vi "ADCS.UnlockECUSecurity.vi"(6 "Diagnostic Protocol":T3, 7 "Addon Name":string, 8 "error in (no error)":errorcluster, 9 "MasterKey":string, 10 "Security":T1={"Type"=enum."None", "Source DLL Path"=path "", "Target DLL Path"=path "", "Security Level"=1, "Static Master Key"="", "Max Key Length"=1, "Host IP Address"="", "ECU  Variant"=0, "Optional Parameter"=0}, 11 "diag ref in":T4={"Diag CAN Handle"=0, "Transport Protocol"=enum."ISO TP - Normal Mode", "Receive Address Extension"=0, "Transmit Address Extension"=0, "Receive CAN Id"=0, "Transmit CAN Id"=0, "Log Frames ?"=FALSE, "My TP Address"=0, "Other TP Address"=0, "T1"=0, "T2"=0, "T3"=0, "T4"=0, "Tx SN"=0, "Block Size"=0, "Rx SN"=0, "VW TP Initialized?"=FALSE, "Tx block no"=0, "baud rate"=0, "Interface"="", "Channel Diag CAN Handle"=0, "UDP Connection ID"=refnum, "TCP Connection ID"=refnum, "Target IP Addr"=0, "Source Address"=0, "Target Address"=0, "Send Header NACK?"=FALSE, "DLL Handle"=0, "NAD"=0, "Time Stamp read first"=0.0, "Time Stamp read last"=0.0, "Time Stamp write first"=0.0, "Time Stamp write last"=0.0, "Time Stamp write"=0.0, "Time Stamp read"=0.0, " I/O Mode"=0, "FD Baudrate"=0, "TX_DL"=8, "RX_DL"=8, "DoIP Protocol Version"=1, " Selected I/O Mode"=0, "TesterPresent Counter"=0, "TesterPresent Limit"=0, "TesterPresent Tick[ms]"=10, "TesterPresent RequireResponse?"=FALSE, "TesterPresent Stored Ref?"=FALSE, "TesterPresent Message"=[], "TesterPresent Task Handle"=0, "TesterPresent Semaphore"=refnum, "Response Plausibility Check"=1, "Default Version?"=TRUE, "Diagostic Globals"={"Timeout FC (Bs)"=250, "Timeout CF (Cr)"=250, "Timeout Diag Command"=1000, "Receive Block Size (BS)"=0, "Wait Time CF (STmin)"=5, "Max Waits (N_WFTmax)"=10, "Waits to Send (N_WAIT)"=0, "Time between Waits (TW)"=25, "Fill CAN Frames?"=TRUE, "Fill Byte"=255, "Invalid Response as Error?"=FALSE, "Max RspPending Count"=5, "VWTP Command Timeout"=50, "Transport Protocol"=enum."Diagnostics on IP", "Diag CAN Handle"=0, "DLL Handle"=0, "Timeout RspPending"=1000}, "Session-based Properties?"=FALSE} {"Diagostic Globals"."Fill Byte" format="%x"; "TesterPresent Message" format="%.0x"; "Selected I/O Mode" items=["CAN", "CAN FD", "CAN FD+BRS", "ECU Determined"]; "DoIP Protocol Version" items=["2010"=1, "2012"=2]; "RX_DL" items=["8"=8, "12"=12, "16"=16, "20"=20, "24"=24, "32"=32, "48"=48, "64"=64]; "TX_DL" items=["8"=8, "12"=12, "16"=16, "20"=20, "24"=24, "32"=32, "48"=48, "64"=64]; "I/O Mode" items=["CAN", "CAN FD", "CAN FD+BRS", "Not yet determined"]}) -> (0 "error out":errorcluster, 1 "success?":bool, 3 "diag ref out":T4={"Diag CAN Handle"=0, "Transport Protocol"=enum."ISO TP - Normal Mode", "Receive Address Extension"=0, "Transmit Address Extension"=0, "Receive CAN Id"=0, "Transmit CAN Id"=0, "Log Frames ?"=FALSE, "My TP Address"=0, "Other TP Address"=0, "T1"=0, "T2"=0, "T3"=0, "T4"=0, "Tx SN"=0, "Block Size"=0, "Rx SN"=0, "VW TP Initialized?"=FALSE, "Tx block no"=0, "baud rate"=0, "Interface"="", "Channel Diag CAN Handle"=0, "UDP Connection ID"=refnum, "TCP Connection ID"=refnum, "Target IP Addr"=0, "Source Address"=0, "Target Address"=0, "Send Header NACK?"=FALSE, "DLL Handle"=0, "NAD"=0, "Time Stamp read first"=0.0, "Time Stamp read last"=0.0, "Time Stamp write first"=0.0, "Time Stamp write last"=0.0, "Time Stamp write"=0.0, "Time Stamp read"=0.0, " I/O Mode"=0, "FD Baudrate"=0, "TX_DL"=8, "RX_DL"=8, "DoIP Protocol Version"=1, " Selected I/O Mode"=0, "TesterPresent Counter"=0, "TesterPresent Limit"=0, "TesterPresent Tick[ms]"=10, "TesterPresent RequireResponse?"=FALSE, "TesterPresent Stored Ref?"=FALSE, "TesterPresent Message"=[], "TesterPresent Task Handle"=0, "TesterPresent Semaphore"=refnum, "Response Plausibility Check"=1, "Default Version?"=TRUE, "Diagostic Globals"={"Timeout FC (Bs)"=250, "Timeout CF (Cr)"=250, "Timeout Diag Command"=1000, "Receive Block Size (BS)"=0, "Wait Time CF (STmin)"=5, "Max Waits (N_WFTmax)"=10, "Waits to Send (N_WAIT)"=0, "Time between Waits (TW)"=25, "Fill CAN Frames?"=TRUE, "Fill Byte"=255, "Invalid Response as Error?"=FALSE, "Max RspPending Count"=5, "VWTP Command Timeout"=50, "Transport Protocol"=enum."Diagnostics on IP", "Diag CAN Handle"=0, "DLL Handle"=0, "Timeout RspPending"=1000}, "Session-based Properties?"=FALSE} {"Diagostic Globals"."Fill Byte" format="%x"; "TesterPresent Message" format="%.0x"; "Selected I/O Mode" items=["CAN", "CAN FD", "CAN FD+BRS", "ECU Determined"]; "DoIP Protocol Version" items=["2010"=1, "2012"=2]; "RX_DL" items=["8"=8, "12"=12, "16"=16, "20"=20, "24"=24, "32"=32, "48"=48, "64"=64]; "TX_DL" items=["8"=8, "12"=12, "16"=16, "20"=20, "24"=24, "32"=32, "48"=48, "64"=64]; "I/O Mode" items=["CAN", "CAN FD", "CAN FD+BRS", "Not yet determined"]})   [LabVIEW 2019, in "Diagnostics Addon Engine.lvlib"]
uses:
  Diagnostics Addon Engine.lvlib
  <vilib>/Automotive Diagnostic Command Set/Diagnostic Transport.llb/Diag Reference.ctl
  <vilib>/Automotive Diagnostic Command Set/Diagnostic Transport.llb/Transport Protocol Selector.ctl
  <vilib>/Automotive Diagnostic Command Set/Diagnostic Transport.llb/DoIP Protocol Version.ctl
  <vilib>/Automotive Diagnostic Command Set/Diagnostic Transport.llb/Diag Globals.ctl
  Addon Shared/Types/Protocol.ctl
  Addon Shared/Types/Security.ctl
  Addon Shared/Types/Security.Type.ctl
  <vilib>/NI/STM/Write Meta Data.vi
  <vilib>/NI/STM/TCP/Write Meta Data (TCP Ref).vi
  <vilib>/NI/STM/Get Connection Reference.vi
  <vilib>/NI/STM/TCP/Get Connection Reference (TCP).vi
  <vilib>/Automotive Diagnostic Command Set/Diagnostic Transport.llb/Diagnostic Service.vi
  <vilib>/Automotive Diagnostic Command Set/Diagnostic Transport.llb/Apply Success Failure Error.vi
  <vilib>/NI/STM/TCP/Write Meta Data (TCP Clst).vi
  <vilib>/NI/NI VeriStand Addon Network Comm/Shared/Comm Send and Receive.vi
  <vilib>/Utility/error.llb/Error Cluster From Error Code.vi
  <vilib>/Utility/SystemLogging/Write to System Log.vi
  Support Libraries/GMLAN/_SubVIs/SecurityAccess_requestSeed.vi
  Support Libraries/GMLAN/_SubVIs/SecurityAccess_sendKey.vi
  Support Libraries/GMLAN/GMLAN.lvlib
  <vilib>/addons/Automotive Diagnostic Command Set/NI_Automotive Diagnostic Command Set.lvlib
  Addon Shared/Diagnostics Addon Shared.lvlib
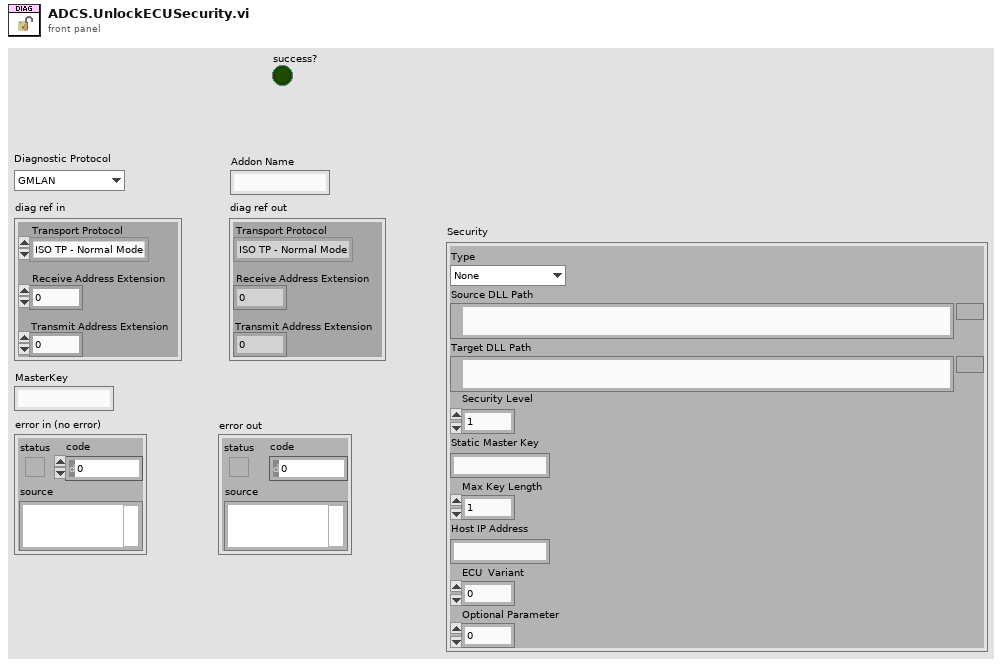
[diagram p1: front panel]
types:
  T1 = typedef "Diagnostics Addon Shared.lvlib/Security.ctl" = cluster{"Type":T2, "Source DLL Path":path, "Target DLL Path":path, "Security Level":u32, "Static Master Key":string, "Max Key Length":u32, "Host IP Address":string, "ECU  Variant":i8, "Optional Parameter":i8}
  T2 = typedef "Diagnostics Addon Shared.lvlib/Security.Type.ctl" = enum16{"None", "SeedKey DLL", "MasterKey (Channel)", "MasterKey (Static)", "SeedKey DLL (Windows)"}
  T3 = typedef "Diagnostics Addon Shared.lvlib/Protocol.ctl" = enum16{"GMLAN", "KWP-2000", "UDS", "User-Defined"}
  T4 = typedef "NI_Automotive Diagnostic Command Set.lvlib/Diag Reference.ctl" = cluster{"Diag CAN Handle":u32, "Transport Protocol":T5, "Receive Address Extension":u8, "Transmit Address Extension":u8, "Receive CAN Id":u32, "Transmit CAN Id":u32, "Log Frames ?":bool, "My TP Address":u8, "Other TP Address":u8, "T1":u16, "T2":u16, "T3":u16, "T4":u16, "Tx SN":u8, "Block Size":u8, "Rx SN":u8, "VW TP Initialized?":bool, "Tx block no":u8, "baud rate":u64, "Interface":string, "Channel Diag CAN Handle":u32, "UDP Connection ID":refnum<k16>, "TCP Connection ID":refnum<k5>, "Target IP Addr":u32, "Source Address":u16, "Target Address":u16, "Send Header NACK?":bool, "DLL Handle":u32, "NAD":u8, "Time Stamp read first":dbl, "Time Stamp read last":dbl, "Time Stamp write first":dbl, "Time Stamp write last":dbl, "Time Stamp write":dbl, "Time Stamp read":dbl, " I/O Mode":u32, "FD Baudrate":u64, "TX_DL":u16, "RX_DL":u16, "DoIP Protocol Version":T6, " Selected I/O Mode":u32, "TesterPresent Counter":u32, "TesterPresent Limit":u32, "TesterPresent Tick[ms]":i32, "TesterPresent RequireResponse?":bool, "TesterPresent Stored Ref?":bool, "TesterPresent Message":u8[], "TesterPresent Task Handle":i32, "TesterPresent Semaphore":T7, "Response Plausibility Check":u32, "Default Version?":bool, "Diagostic Globals":T8, "Session-based Properties?":bool}
  T5 = typedef "NI_Automotive Diagnostic Command Set.lvlib/Transport Protocol Selector.ctl" = enum16{"ISO TP - Normal Mode", "ISO TP - Mixed Mode", "VW TP 2.0", "Diagnostics on IP", "ISO TP LIN"}
  T6 = typedef "NI_Automotive Diagnostic Command Set.lvlib/DoIP Protocol Version.ctl" = u8
  T7 = typedef "Semaphore RefNum" = refnum<k1>
  T8 = typedef "NI_Automotive Diagnostic Command Set.lvlib/Diag Globals.ctl" = cluster{"Timeout FC (Bs)":u32, "Timeout CF (Cr)":u32, "Timeout Diag Command":u32, "Receive Block Size (BS)":u8, "Wait Time CF (STmin)":u8, "Max Waits (N_WFTmax)":u8, "Waits to Send (N_WAIT)":i32, "Time between Waits (TW)":u32, "Fill CAN Frames?":bool, "Fill Byte":u32, "Invalid Response as Error?":bool, "Max RspPending Count":u32, "VWTP Command Timeout":u32, "Transport Protocol":T5, "Diag CAN Handle":u32, "DLL Handle":u32, "Timeout RspPending":u32}
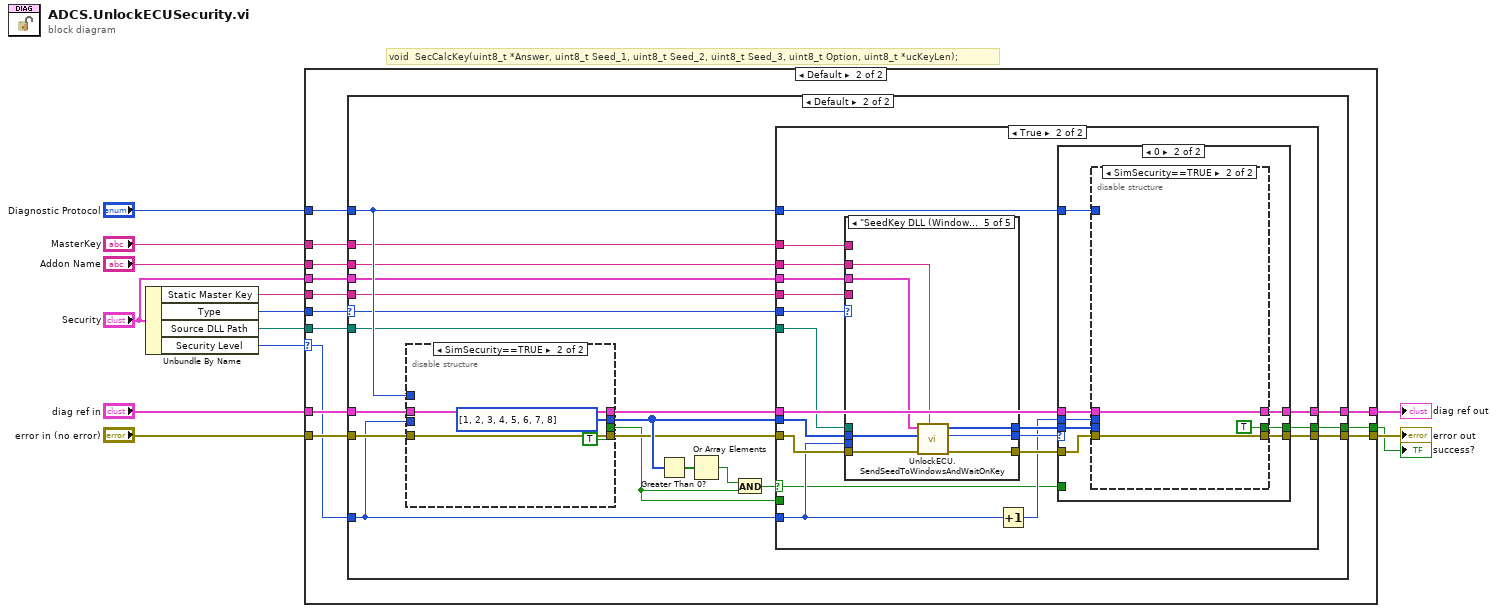
[diagram p0: block diagram]
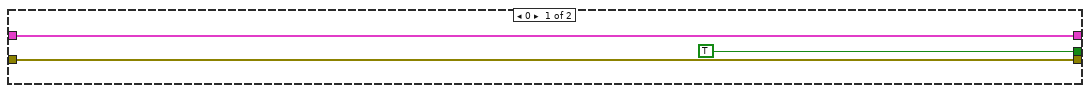
[diagram p2: hidden frame]
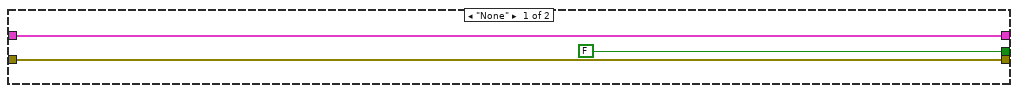
[diagram p3: hidden frame]
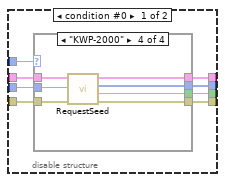
[diagram p4: hidden frame]
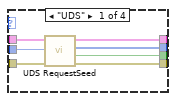
[diagram p5: hidden frame]
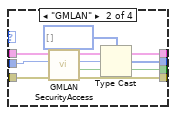
[diagram p6: hidden frame]
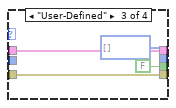
[diagram p7: hidden frame]
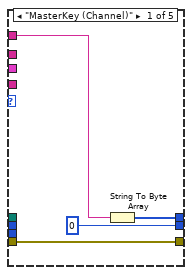
[diagram p9: hidden frame]
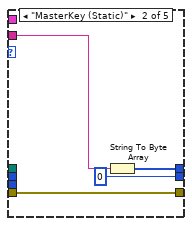
[diagram p10: hidden frame]
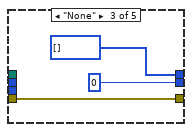
[diagram p11: hidden frame]
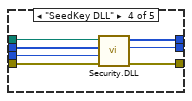
[diagram p12: hidden frame]
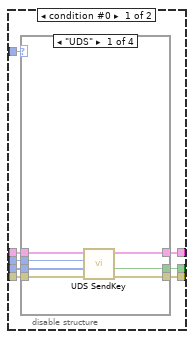
[diagram p14: hidden frame]
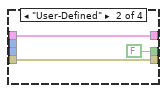
[diagram p15: hidden frame]
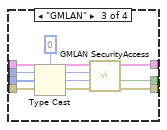
[diagram p16: hidden frame]
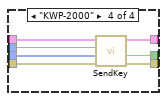
[diagram p17: hidden frame]
diagram:
  # "void  SecCalcKey(uint8_t *Answer, uint8_t Seed_1, uint8_t Seed_2, uint8_t Seed_3, uint8_t Option, uint8_t *ucKeyLen);"
  n1 = Unbundle By Name("Security") -> ("Static Master Key"=w3:string, "Type"=w5:T2, "Source DLL Path"=w8:path, "Security Level"=w7:u32)
  n2 = case shown="Default" w7 {
    selector: w7 -> [_ w23]
    tunnel: "diag ref in" -> [w16 w29]
    tunnel: [w16 w28] -> w12
    tunnel: "Diagnostic Protocol" -> [_ w27]
    tunnel: "error in (no error)" -> [w15 w26]
    tunnel: [w15 w25] -> w9
    tunnel: w8 -> [_ w24]
    tunnel: [TRUE ("success?") w22] -> w6
    tunnel: w5 -> [_ w21]
    tunnel: "MasterKey" -> [_ w20]
    tunnel: w3 -> [_ w19]
    tunnel: "Security" -> [_ w18]
    tunnel: "Addon Name" -> [_ w17]
    frame 0 {
    }
    frame Default {
      n3 = case shown="Default" w21 {
        selector: w21 -> [_ w37]
        tunnel: w29 -> [w32 w52]
        tunnel: [w32 w51] -> w28
        tunnel: w27 -> [_ w47]
        tunnel: w26 -> [w31 w44]
        tunnel: [w31 w42] -> w25
        tunnel: w24 -> [_ w41]
        tunnel: w23 -> [_ w40]
        tunnel: [FALSE ("success?") w38] -> w22
        tunnel: w20 -> [_ w36]
        tunnel: w19 -> [_ w35]
        tunnel: w18 -> [_ w34]
        tunnel: w17 -> [_ w33]
        frame "None" {
        }
        frame Default {
          n4 = disable-structure shown="SimSecurity==TRUE" {
            disable-tunnel: w52 -> [w60 w90]
            disable-tunnel: w47 -> [w59 _]
            disable-tunnel: [w58 w90] -> w46
            disable-tunnel: [w57 u8[] [1, 2, 3, 4, 5, 6, 7, 8] ("seed out")] -> w45
            disable-tunnel: w44 -> [w56 w91]
            disable-tunnel: [w55 w91] -> w43
            disable-tunnel: w40 -> [w54 _]
            disable-tunnel: [w53 TRUE ("success?")] -> w39
            frame condition #0 {
              n5 = case shown="\"KWP-2000\"" w59 {
                tunnel: w56 -> [w64 w74 w80 w87]
                tunnel: w60 -> [w65 w76 w79 w86]
                tunnel: [w61 w71 w79 w85] -> w58
                tunnel: w54 -> [w66 w75 _ w84]
                tunnel: [w63 w73 w80 w83] -> w55
                tunnel: [w62 w68 u8[] [] ("seed out") w82] -> w57
                tunnel: [w67 w72 FALSE ("success?") w81] -> w53
                frame "UDS" {
                  n6 = call <vilib>:"UDS RequestSeed.vi"("error in (no error)"=w64, "access mode"=w66, "diag ref in"=w65) -> ("error out"=w63:errorcluster, "success?"=w67:bool, "seed out"=w62:u8[], "diag ref out"=w61:T4)  [unwired: 5 in]
                }
                frame "GMLAN" {
                  n7 = call-poly "GMLAN SecurityAccess.vi"("error in (no error)"=w74, "subFunction"=w75, "diag ref in"=w76) -> ("error out"=w73:errorcluster, "success?"=w72:bool, "SecuritySeed"=w70:u16, "diag ref out"=w71:T4)  [unwired: 5 in]
                  n8 = Type Cast(type=u8[] [] ("seed out"), x=w70) -> (*(type *) &x=w68:u8[])
                }
                frame "User-Defined" {
                }
                frame "KWP-2000" {
                  n9 = call <vilib>:"RequestSeed.vi"("error in (no error)"=w87, "access mode"=w84, "diag ref in"=w86) -> ("error out"=w83:errorcluster, "success?"=w81:bool, "seed out"=w82:u8[], "diag ref out"=w85:T4)  [unwired: 5 in]
                }
              }
            }
            frame condition #1 (active) {
            }
          }
          n10 = Greater Than 0?(x=w45) -> (x > 0?=w50:bool[])
          n11 = Or Array Elements(Boolean array=w50) -> (logical OR=w48:bool)
          n12 = And(x=w48, y=w39) -> (x .and. y?=w49:bool)
          n13 = case shown="True" w49 {
            selector: w49 -> [_ w101]
            tunnel: [w93 w113] -> w42
            tunnel: w41 -> [_ w107]
            tunnel: w46 -> [w94 w112]
            tunnel: w45 -> [_ w108]
            tunnel: w43 -> [w93 w109]
            tunnel: [w94 w111] -> w51
            tunnel: w40 -> [_ w103]
            tunnel: w47 -> [_ w110]
            tunnel: [w92 w100] -> w38
            tunnel: w39 -> [w92 _]
            tunnel: w37 -> [_ w99]
            tunnel: w36 -> [_ w98]
            tunnel: w35 -> [_ w97]
            tunnel: w34 -> [_ w96]
            tunnel: w33 -> [_ w95]
            frame False {
              # "Positive Response - No Seed\n                   or\nNegative Response"
            }
            frame True {
              n14 = case shown="\"SeedKey DLL (Windows)\"" w99 {
                tunnel: w109 -> [w116 w120 w124 w131 w138]
                tunnel: w108 -> [_ _ _ w130 w134]
                tunnel: w107 -> [_ _ _ w129 _]
                tunnel: [w117 w121 u8[] [] ("unsigned byte array") w128 w135] -> w106
                tunnel: [u8 0 ("lockstatus") u8 0 ("lockstatus") u8 0 ("lockstatus") w127 w137] -> w105
                tunnel: [w116 w120 w124 w126 w136] -> w104
                tunnel: w103 -> [_ _ _ w125 _]
                tunnel: w98 -> [w114 _ _ _ _]
                tunnel: w97 -> [_ w118 _ _ _]
                tunnel: w96 -> [_ _ _ _ w133]
                tunnel: w95 -> [_ _ _ _ w132]
                frame "MasterKey (Channel)" {
                  n15 = String To Byte Array(string=w114) -> (unsigned byte array=w117:u8[])
                }
                frame "MasterKey (Static)" {
                  n16 = String To Byte Array(string=w118) -> (unsigned byte array=w121:u8[])
                }
                frame "None" {
                }
                frame "SeedKey DLL" {
                  n17 = call "Security.DLL.vi"("error in (no error)"=w131, "Option"=w125, "Seed"=w130, "path in"=w129) -> ("error out"=w126:errorcluster, "lockstatus"=w127:u8, "unsigned byte array"=w128:u8[])  [unwired: 5 in]
                }
                frame "SeedKey DLL (Windows)" {
                  n18 = call "UnlockECU.SendSeedToWindowsAndWaitOnKey.vi"("Addon Name"=w132, "error in (no error)"=w138, "Seed"=w134, "Security"=w133) -> ("error out"=w136:errorcluster, "Error code"=w137:i32, "Key"=w135:u8[])  [unwired: 5 in]
                }
              }
              n19 = Increment(x=w103) -> (x+1=w102:u32)
              n20 = case shown="0" w105 {
                tunnel: [w141 w149] -> w113
                tunnel: w112 -> [w140 w148]
                tunnel: [w140 w147] -> w111
                tunnel: w102 -> [_ w146]
                tunnel: w110 -> [_ w145]
                tunnel: w104 -> [w141 w144]
                tunnel: w106 -> [_ w143]
                tunnel: [w139 w142] -> w100
                tunnel: w101 -> [w139 _]
                frame Default {
                }
                frame 0 {
                  n21 = disable-structure shown="SimSecurity==TRUE" {
                    disable-tunnel: [w157 w186] -> w149
                    disable-tunnel: w148 -> [w156 w185]
                    disable-tunnel: [w155 w185] -> w147
                    disable-tunnel: w146 -> [w154 _]
                    disable-tunnel: w145 -> [w153 _]
                    disable-tunnel: w144 -> [w152 w186]
                    disable-tunnel: w143 -> [w151 _]
                    disable-tunnel: [w150 TRUE ("success?")] -> w142
                    frame condition #0 {
                      n22 = case shown="\"UDS\"" w153 {
                        tunnel: [w162 w167 w173 w183] -> w157
                        tunnel: w156 -> [w164 w166 w175 w182]
                        tunnel: w152 -> [w161 w167 w174 w181]
                        tunnel: [w163 w166 w172 w180] -> w155
                        tunnel: w154 -> [w159 _ w176 w179]
                        tunnel: w151 -> [w160 _ w171 w178]
                        tunnel: [w158 FALSE ("success?") w168 w177] -> w150
                        frame "UDS" {
                          n23 = call <vilib>:"UDS SendKey.vi"("error in (no error)"=w161, "key in"=w160, "access mode"=w159, "diag ref in"=w164) -> ("error out"=w162:errorcluster, "success?"=w158:bool, "diag ref out"=w163:T4)  [unwired: 5 in]
                        }
                        frame "User-Defined" {
                        }
                        frame "GMLAN" {
                          n24 = Type Cast(type=u16 0 ("SecuritySeed"), x=w171) -> (*(type *) &x=w170:u16)
                          n25 = call-poly "GMLAN SecurityAccess.vi"("error in (no error)"=w174, "SecuritySeed"=w170, "subFunction"=w176, "diag ref in"=w175) -> ("error out"=w173:errorcluster, "success?"=w168:bool, "diag ref out"=w172:T4)  [unwired: 5 in]
                        }
                        frame "KWP-2000" {
                          n26 = call <vilib>:"SendKey.vi"("error in (no error)"=w181, "key in"=w178, "access mode"=w179, "diag ref in"=w182) -> ("error out"=w183:errorcluster, "success?"=w177:bool, "diag ref out"=w180:T4)  [unwired: 5 in]
                        }
                      }
                    }
                    frame condition #1 (active) {
                    }
                  }
                }
              }
            }
          }
        }
      }
    }
  }
  "error out" <- w9
  "diag ref out" <- w12
  "success?" <- w6
